vi "CcsCSV2Cluster.vi"(8 "error in (no error)":errorcluster, 11 "CCSPath":path) -> (0 "error out":errorcluster, 3 "AllDataArrays":T1 {"DataAnlysisArray"."Time" format="%.6f"; "DataAnlysisArray"."TimeStamp" format="%^<%.3X\n%x>T"; "DUTDataArray"."TimeStamp" format="%^<%.3X\n%x>T"; "DUTDataArray"."Time" format="%.6f"; "NIDataArray"."TimeStamp" format="%^<%.3X\n%x>T"; "NIDataArray"."Time" format="%.6f"})   [LabVIEW 2014]
uses:
  typedefs/NICalcAnalysis.ctl
  typedefs/CalcPhasorError.ctl
  typedefs/DUTData.ctl
  typedefs/PhasorRectangular.ctl
  typedefs/NIData.ctl
  typedefs/NISTData.ctl
  typedefs/NIDataArray.ctl
  <vilib>/Utility/file.llb/Read From Spreadsheet File (string).vi
panel:
  out "Numeric 3":i32
  out "Numeric 2":i32
  out "Numeric":i32
  in  "RefDataCluster":T3 {"TimeStamp" format="%^<%.3X\n%x>T"; "Time" format="%.6f"}
  in  "PmuDataCluster":T5 {"TimeStamp" format="%^<%.3X\n%x>T"; "Time" format="%.6f"}
  in  "NICalcAnalysis":T6 {"Time" format="%.6f"; "TimeStamp" format="%^<%.3X\n%x>T"}
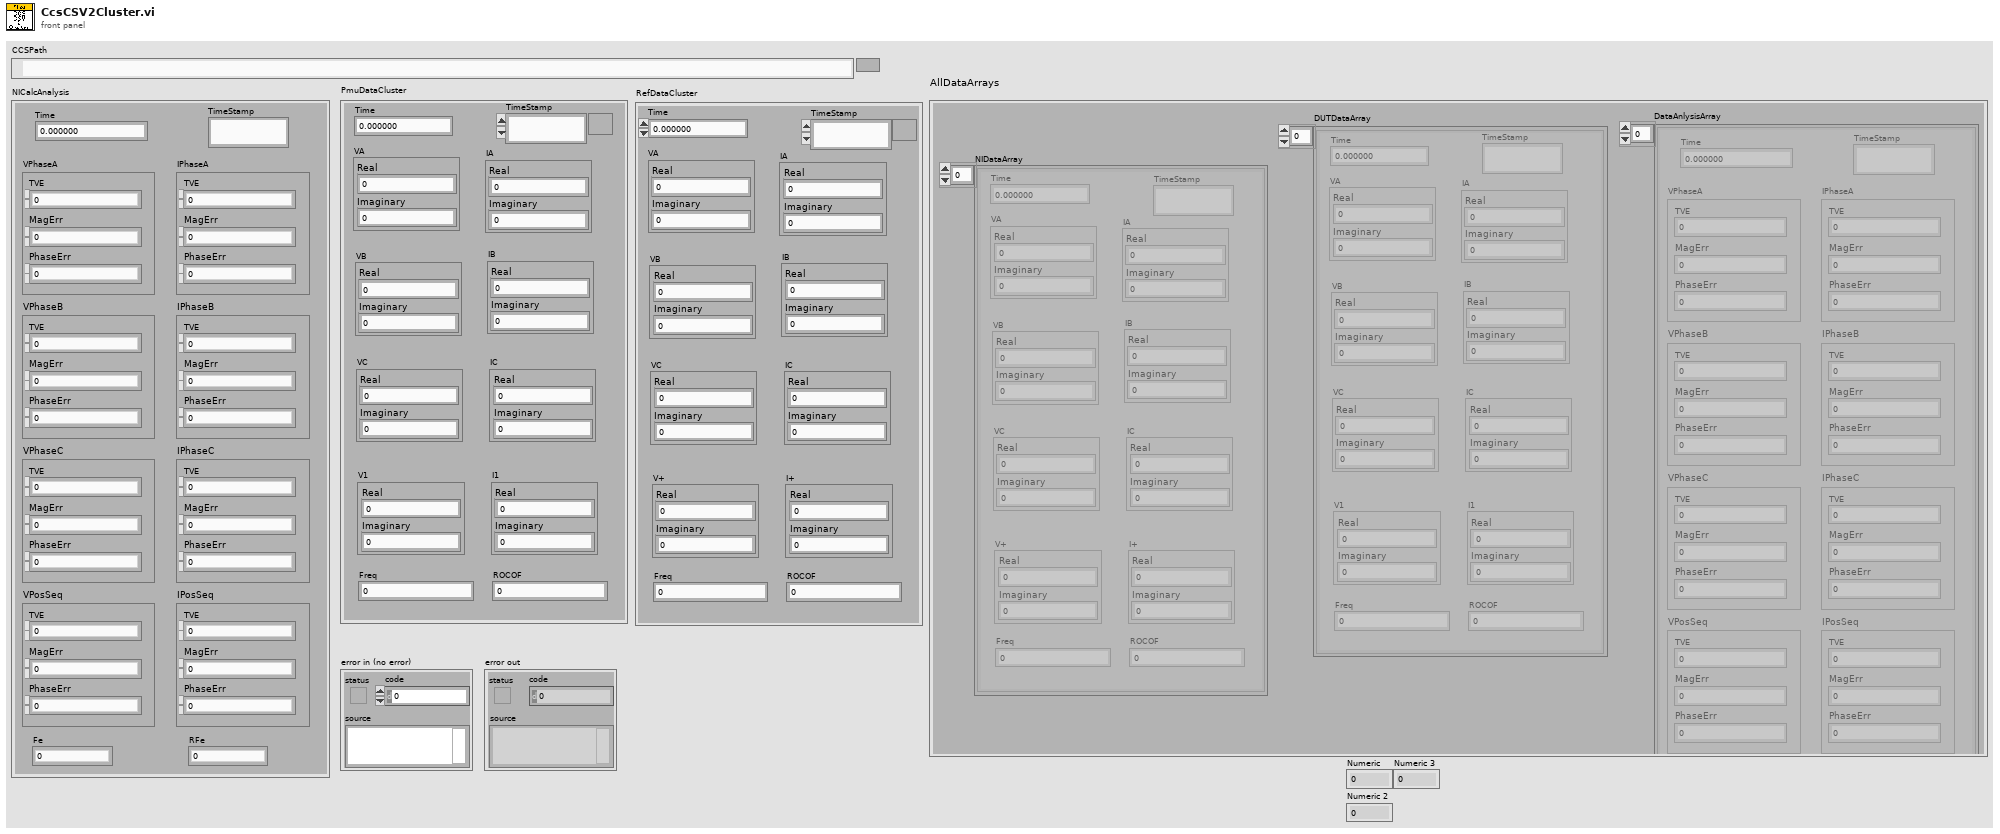
[diagram p1: front panel]
types:
  T1 = typedef "NISTData.ctl" = cluster{"NIDataArray":T2, "DUTDataArray":T5[], "DataAnlysisArray":T6[]}
  T2 = typedef "NIDataArray.ctl" = T3[]
  T3 = typedef "NIData.ctl" = cluster{"Time":dbl, "VA":T4, "VB":T4, "VC":T4, "V+":T4, "IA":T4, "IB":T4, "IC":T4, "I+":T4, "Freq":dbl, "ROCOF":dbl, "TimeStamp":timestamp}
  T4 = typedef "PhasorRectangular.ctl" = cluster{"Real":dbl, "Imaginary":dbl}
  T5 = typedef "DUTData.ctl" = cluster{"Time":dbl, "VA":T4, "VB":T4, "VC":T4, "V1":T4, "IA":T4, "IB":T4, "IC":T4, "I1":T4, "Freq":dbl, "ROCOF":dbl, "TimeStamp":timestamp}
  T6 = typedef "NICalcAnalysis.ctl" = cluster{"Time":dbl, "VPhaseA":T7, "VPhaseB":T7, "VPhaseC":T7, "VPosSeq":T7, "IPhaseA":T7, "IPhaseB":T7, "IPhaseC":T7, "IPosSeq":T7, "Fe":dbl, "RFe":dbl, "TimeStamp":timestamp}
  T7 = typedef "CalcPhasorError.ctl" = cluster{"TVE":dbl, "MagErr":dbl, "PhaseErr":dbl}
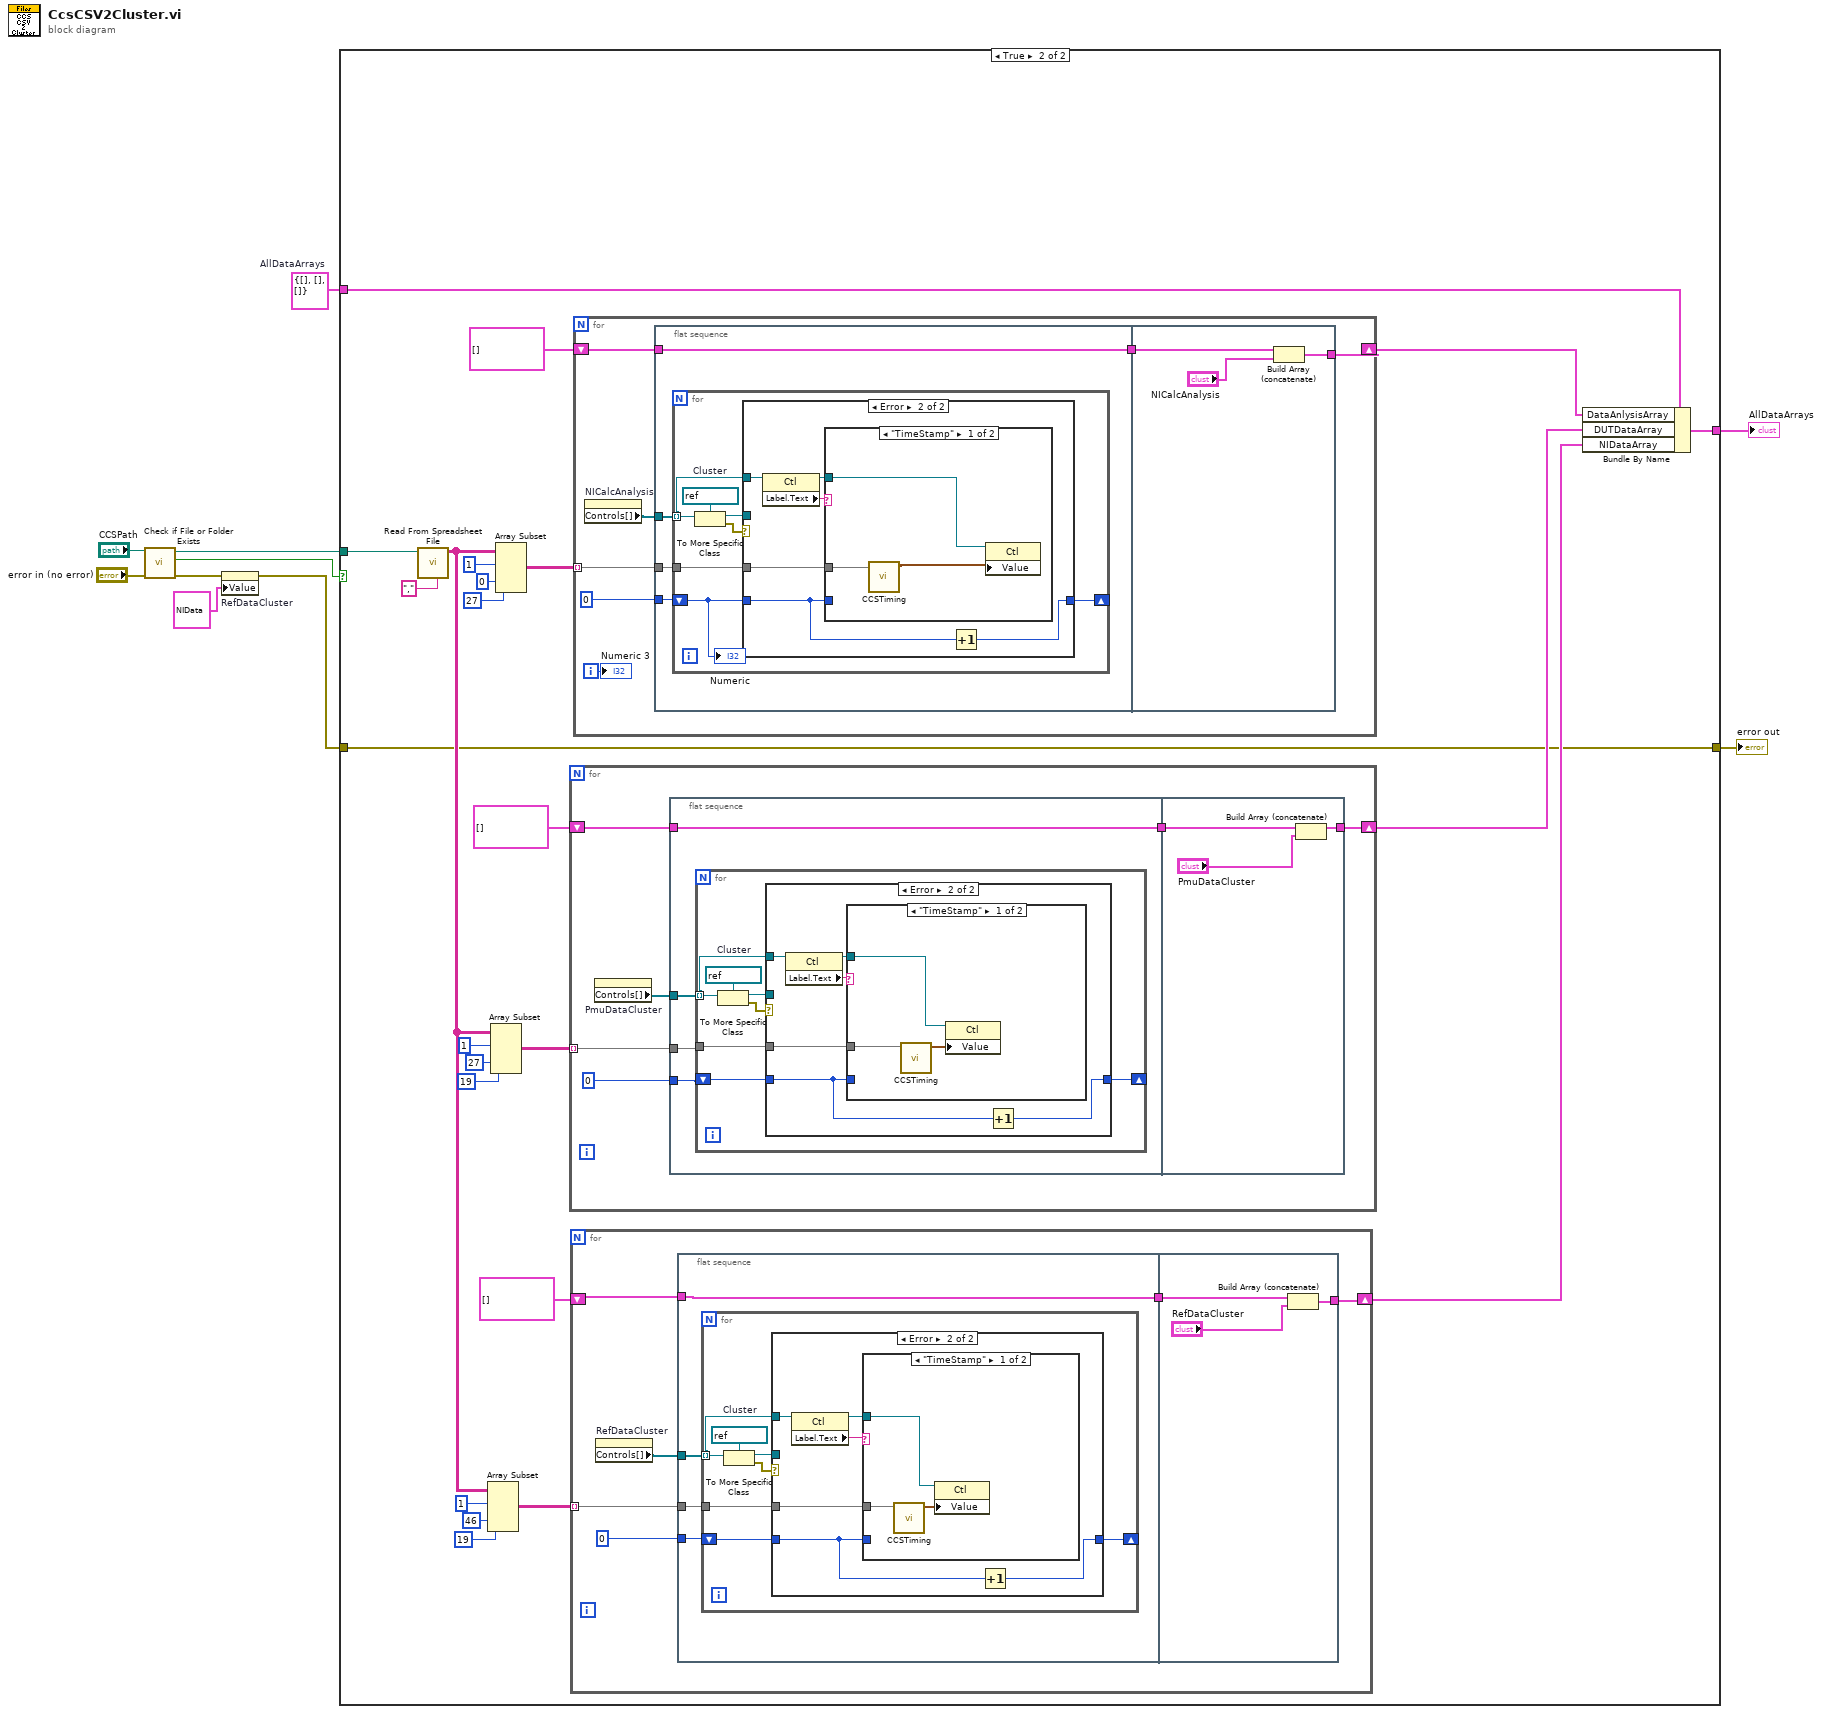
[diagram p0: block diagram]
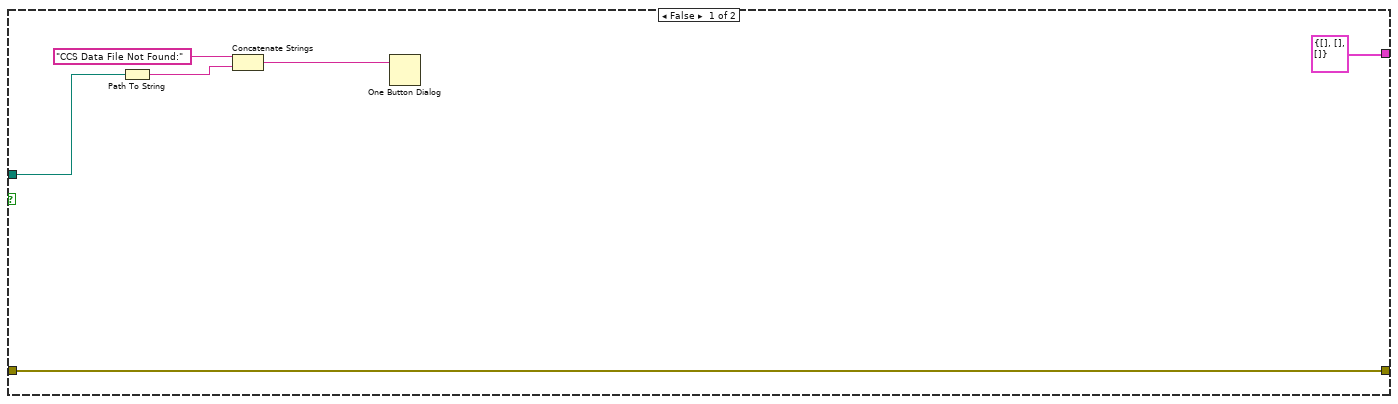
[diagram p2: hidden frame]
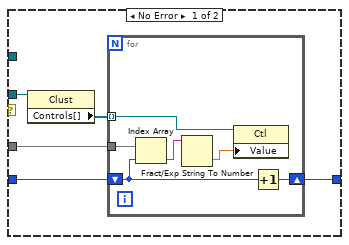
[diagram p3: hidden frame]
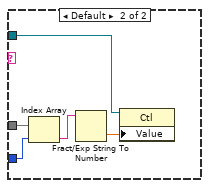
[diagram p4: hidden frame]
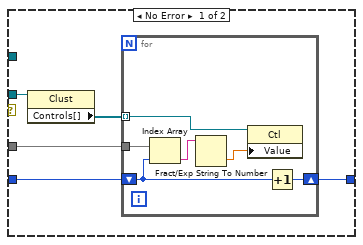
[diagram p5: hidden frame]
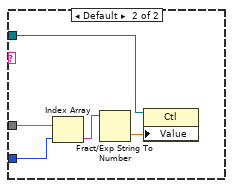
[diagram p6: hidden frame]
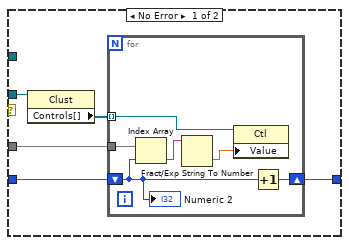
[diagram p7: hidden frame]
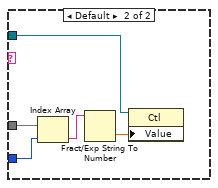
[diagram p8: hidden frame]
diagram:
  w4 = T1 {"NIDataArray"=[], "DUTDataArray"=[], "DataAnlysisArray"=[]}  # AllDataArrays
  n1 = call <vilib>:"Check if File or Folder Exists.vi"("error in (no error)"="error in (no error)", "path"="CCSPath") -> ("error out"=w3:errorcluster, "file or folder exists?"=w7:bool, "dup path"=w8:path)  [unwired: 7 in]
  n2 = property on="RefDataCluster" class="Clust (strict)"(error in=w3, "Value"=T3 {"Time"=0.0, "VA"={"Real"=0.0, "Imaginary"=0.0}, "VB"={"Real"=0.0, "Imaginary"=0.0}, "VC"={"Real"=0.0, "Imaginary"=0.0}, "V+"={"Real"=0.0, "Imaginary"=0.0}, "IA"={"Real"=0.0, "Imaginary"=0.0}, "IB"={"Real"=0.0, "Imaginary"=0.0}, "IC"={"Real"=0.0, "Imaginary"=0.0}, "I+"={"Real"=0.0, "Imaginary"=0.0}, "Freq"=0.0, "ROCOF"=0.0, "TimeStamp"=timestamp(0 s since 1904-01-01)}) -> (error out=w2:errorcluster)  [unwired: 1 in, 1 out]
  n3 = case shown="True" w7 {
    tunnel: w8 -> [w14 w18]
    tunnel: w2 -> [w12 w22]
    tunnel: [T1 {"NIDataArray"=[], "DUTDataArray"=[], "DataAnlysisArray"=[]} ("AllDataArrays") w23] -> w6
    tunnel: [w12 w22] -> w5
    tunnel: w4 -> [_ w21]
    frame False {
      n4 = Path To String(path=w14) -> (string=w15:string)
      n5 = Concatenate Strings("CCS Data File Not Found:", w15) -> (w13:string)
      n6 = One Button Dialog(message=w13) -> ()  [unwired: 1 in, 1 out]
    }
    frame True {
      n7 = call-poly <vilib>:"Read From Spreadsheet File.vi"("delimiter (\\t)"="," ("delimiter (\\t)"), "file path (dialog if empty)"=w18) -> ("all rows"=w27:string[][])  [unwired: 5 in, 4 out]
      n8 = Array Subset(array=w27, index (row)=1 ("index"), index (col)=46 ("index"), length (col)=19 ("length")) -> (w28:string[][])  [unwired: 1 in]
      n9 = Array Subset(array=w27, index (row)=1 ("index"), index (col)=27 ("index"), length (col)=19 ("length")) -> (w35:string[][])  [unwired: 1 in]
      n10 = Array Subset(array=w27, index (row)=1 ("index"), index (col)=0 ("index"), length (col)=27 ("length")) -> (w36:string[][])  [unwired: 1 in]
      n11 = for {
        tunnel: w35 -> [w90] mode=indexing
        shift-right: [w88] -> w25
        shift-left: T5[] [] -> [w87]
        n12 = property on="PmuDataCluster" class="Clust (strict)"() -> ("Controls[]"=w91:refnum<vi>[])  [unwired: 2 in, 2 out]
        n13 = flat-sequence {
          tunnel: w91 -> [w95]
          tunnel: w90 -> [w94]
          tunnel: 0 ("index") -> [w93]
          tunnel: w87 -> [w92]
          tunnel: [w92] -> w86
          tunnel: [w130] -> w88
          tunnel: w86 -> [w129]
          frame #0 {
            n14 = for {
              tunnel: w95 -> [w96] mode=indexing
              tunnel: w94 -> [w99]
              shift-right: [w97] -> _
              shift-left: w93 -> [w98]
              w102 = refnum<vi> refnum  # Cluster
              n15 = To More Specific Class(target class=w102, reference=w96) -> (specific class reference=w100:refnum<vi>, error out=w101:errorcluster)  [unwired: 1 in]
              n16 = case shown="Error" w101 {
                tunnel: w100 -> [w107 _]
                tunnel: w99 -> [w105 w116]
                tunnel: w98 -> [w104 w115]
                tunnel: [w103 w114] -> w97
                tunnel: w96 -> [_ w119]
                frame No Error {
                  n17 = property class="Clust"(reference=w107) -> ("Controls[]"=w106:refnum<vi>[])  [unwired: 1 in, 2 out]
                  n18 = for {
                    tunnel: w106 -> [w110] mode=indexing
                    tunnel: w105 -> [w113]
                    shift-right: [w108] -> w103
                    shift-left: w104 -> [w112]
                    n19 = Index Array(array=w113, index=w112) -> (element=w111:string)
                    n20 = Fract/Exp String To Number(string=w111) -> (number=w109:dbl)  [unwired: 3 in, 1 out]
                    n21 = property class="Ctl"(reference=w110, "Value"=w109) -> ()  [unwired: 1 in, 2 out]
                    n22 = Increment(x=w112) -> (x+1=w108:i32)
                  }
                }
                frame Error {
                  n23 = property class="Ctl"(reference=w119) -> (reference out=w117:refnum<vi>, "Label.Text"=w118:string)  [unwired: 1 in, 1 out]
                  n24 = case shown="\"TimeStamp\"" w118 {
                    tunnel: w117 -> [w122 w124]
                    tunnel: w116 -> [w121 w126]
                    tunnel: w115 -> [_ w127]
                    frame "TimeStamp" {
                      n25 = call "CCSTiming.vi"("array"=w121) -> ("timestamp out"=w120:timestamp)  [unwired: 9 in, 1 out]
                      n26 = property class="Ctl"(reference=w122, "Value"=w120) -> ()  [unwired: 1 in, 2 out]
                    }
                    frame Default {
                      n27 = Index Array(array=w126, index=w127) -> (element=w125:string)
                      n28 = Fract/Exp String To Number(string=w125) -> (number=w123:dbl)  [unwired: 3 in, 1 out]
                      n29 = property class="Ctl"(reference=w124, "Value"=w123) -> ()  [unwired: 1 in, 2 out]
                    }
                  }
                  n30 = Increment(x=w115) -> (x+1=w114:i32)
                }
              }
            }
          }
          frame #1 {
            n31 = Build Array (concatenate)(w129, "PmuDataCluster") -> (w130:T5[])
          }
        }
      }
      n32 = for {
        tunnel: w28 -> [w45] mode=indexing
        shift-right: [w43] -> w24
        shift-left: T3[] [] -> [w42]
        n33 = property on="RefDataCluster" class="Clust (strict)"() -> ("Controls[]"=w46:refnum<vi>[])  [unwired: 2 in, 2 out]
        n34 = flat-sequence {
          tunnel: w46 -> [w50]
          tunnel: w45 -> [w49]
          tunnel: 0 ("index") -> [w48]
          tunnel: w42 -> [w47]
          tunnel: [w47] -> w41
          tunnel: [w85] -> w43
          tunnel: w41 -> [w84]
          frame #0 {
            n35 = for {
              tunnel: w50 -> [w51] mode=indexing
              tunnel: w49 -> [w54]
              shift-right: [w52] -> _
              shift-left: w48 -> [w53]
              w57 = refnum<vi> refnum  # Cluster
              n36 = To More Specific Class(target class=w57, reference=w51) -> (specific class reference=w55:refnum<vi>, error out=w56:errorcluster)  [unwired: 1 in]
              n37 = case shown="Error" w56 {
                tunnel: w55 -> [w62 _]
                tunnel: w54 -> [w60 w71]
                tunnel: w53 -> [w59 w70]
                tunnel: [w58 w69] -> w52
                tunnel: w51 -> [_ w74]
                frame No Error {
                  n38 = property class="Clust"(reference=w62) -> ("Controls[]"=w61:refnum<vi>[])  [unwired: 1 in, 2 out]
                  n39 = for {
                    tunnel: w61 -> [w65] mode=indexing
                    tunnel: w60 -> [w68]
                    shift-right: [w63] -> w58
                    shift-left: w59 -> [w67]
                    n40 = Index Array(array=w68, index=w67) -> (element=w66:string)
                    n41 = Fract/Exp String To Number(string=w66) -> (number=w64:dbl)  [unwired: 3 in, 1 out]
                    n42 = property class="Ctl"(reference=w65, "Value"=w64) -> ()  [unwired: 1 in, 2 out]
                    n43 = Increment(x=w67) -> (x+1=w63:i32)
                  }
                }
                frame Error {
                  n44 = property class="Ctl"(reference=w74) -> (reference out=w72:refnum<vi>, "Label.Text"=w73:string)  [unwired: 1 in, 1 out]
                  n45 = case shown="\"TimeStamp\"" w73 {
                    tunnel: w72 -> [w77 w79]
                    tunnel: w71 -> [w76 w81]
                    tunnel: w70 -> [_ w82]
                    frame "TimeStamp" {
                      n46 = call "CCSTiming.vi"("array"=w76) -> ("timestamp out"=w75:timestamp)  [unwired: 9 in, 1 out]
                      n47 = property class="Ctl"(reference=w77, "Value"=w75) -> ()  [unwired: 1 in, 2 out]
                    }
                    frame Default {
                      n48 = Index Array(array=w81, index=w82) -> (element=w80:string)
                      n49 = Fract/Exp String To Number(string=w80) -> (number=w78:dbl)  [unwired: 3 in, 1 out]
                      n50 = property class="Ctl"(reference=w79, "Value"=w78) -> ()  [unwired: 1 in, 2 out]
                    }
                  }
                  n51 = Increment(x=w70) -> (x+1=w69:i32)
                }
              }
            }
          }
          frame #1 {
            n52 = Build Array (concatenate)(w84, "RefDataCluster") -> (w85:T3[])
          }
        }
      }
      n53 = for {
        tunnel: w36 -> [w137] mode=indexing
        shift-right: [w132] -> w26
        shift-left: T6[] [] -> [w135]
        i -> [w131]
        n54 = property on="NICalcAnalysis" class="Clust (strict)"() -> ("Controls[]"=w134:refnum<vi>[])  [unwired: 2 in, 2 out]
        n55 = flat-sequence {
          tunnel: w137 -> [w141]
          tunnel: 0 ("index") -> [w140]
          tunnel: w135 -> [w138]
          tunnel: w134 -> [w139]
          tunnel: [w138] -> w133
          tunnel: [w176] -> w132
          tunnel: w133 -> [w175]
          frame #0 {
            n56 = for {
              tunnel: w139 -> [w143] mode=indexing
              tunnel: w141 -> [w145]
              shift-right: [w144] -> _
              shift-left: w140 -> [w142]
              w148 = refnum<vi> refnum  # Cluster
              n57 = To More Specific Class(target class=w148, reference=w143) -> (specific class reference=w146:refnum<vi>, error out=w147:errorcluster)  [unwired: 1 in]
              n58 = case shown="Error" w147 {
                tunnel: w146 -> [w153 _]
                tunnel: w145 -> [w151 w162]
                tunnel: w142 -> [w150 w161]
                tunnel: [w149 w160] -> w144
                tunnel: w143 -> [_ w165]
                frame No Error {
                  n59 = property class="Clust"(reference=w153) -> ("Controls[]"=w152:refnum<vi>[])  [unwired: 1 in, 2 out]
                  n60 = for {
                    tunnel: w152 -> [w157] mode=indexing
                    tunnel: w151 -> [w159]
                    shift-right: [w155] -> w149
                    shift-left: w150 -> [w154]
                    n61 = Index Array(array=w159, index=w154) -> (element=w158:string)
                    n62 = Fract/Exp String To Number(string=w158) -> (number=w156:dbl)  [unwired: 3 in, 1 out]
                    n63 = property class="Ctl"(reference=w157, "Value"=w156) -> ()  [unwired: 1 in, 2 out]
                    n64 = Increment(x=w154) -> (x+1=w155:i32)
                    "Numeric 2" <- w154
                  }
                }
                frame Error {
                  n65 = property class="Ctl"(reference=w165) -> (reference out=w163:refnum<vi>, "Label.Text"=w164:string)  [unwired: 1 in, 1 out]
                  n66 = case shown="\"TimeStamp\"" w164 {
                    tunnel: w163 -> [w168 w170]
                    tunnel: w162 -> [w167 w172]
                    tunnel: w161 -> [_ w173]
                    frame "TimeStamp" {
                      n67 = call "CCSTiming.vi"("array"=w167) -> ("timestamp out"=w166:timestamp)  [unwired: 9 in, 1 out]
                      n68 = property class="Ctl"(reference=w168, "Value"=w166) -> ()  [unwired: 1 in, 2 out]
                    }
                    frame Default {
                      n69 = Index Array(array=w172, index=w173) -> (element=w171:string)
                      n70 = Fract/Exp String To Number(string=w171) -> (number=w169:dbl)  [unwired: 3 in, 1 out]
                      n71 = property class="Ctl"(reference=w170, "Value"=w169) -> ()  [unwired: 1 in, 2 out]
                    }
                  }
                  n72 = Increment(x=w161) -> (x+1=w160:i32)
                }
              }
              "Numeric" <- w142
            }
          }
          frame #1 {
            n73 = Build Array (concatenate)(w175, "NICalcAnalysis") -> (w176:T6[])
          }
        }
        "Numeric 3" <- w131
      }
      n74 = Bundle By Name(cluster=w21, "DataAnlysisArray"=w26, "DUTDataArray"=w25, "NIDataArray"=w24) -> (w23:T1)
    }
  }
  "AllDataArrays" <- w6
  "error out" <- w5
